vi "Actor Core.vi"(8 "error in":errorcluster, 11 "ListboxBusMonitorPanel in":refnum<class "ListboxBusMonitorPanel.lvclass">) -> (0 "error out":errorcluster, 3 "Actor out":refnum<class "Actor.lvclass">)   [LabVIEW 2020, in "MVA Framework.lvlib" / "ListboxBusMonitor.lvlib" / "ListboxBusMonitorPanel.lvclass"]
doc: "(<B>Filename</B>: Actor Framework.lvlib:Actor.lvclass:Actor Core.vi)\n\nReceives messages to the actor, reacts to them, and initiates any error handling that may shut the actor down.\n\nDescendant classes may override this VI to append parallel tasks for the actor to complete while it handles messages. Overrides use the Call Parent Method node."
uses:
  ListboxBusMonitorPanel.lvclass
  <vilib>/ActorFramework/Actor/Actor.lvclass
  ListboxBusMonitorPanel.lvclass/ListboxBusMonitorPanel.ctl
  modules/listbox-extensions/Source/ListboxExtensions.lvlib
panel:
  in  "Multicolumn Listbox":i32(listbox)
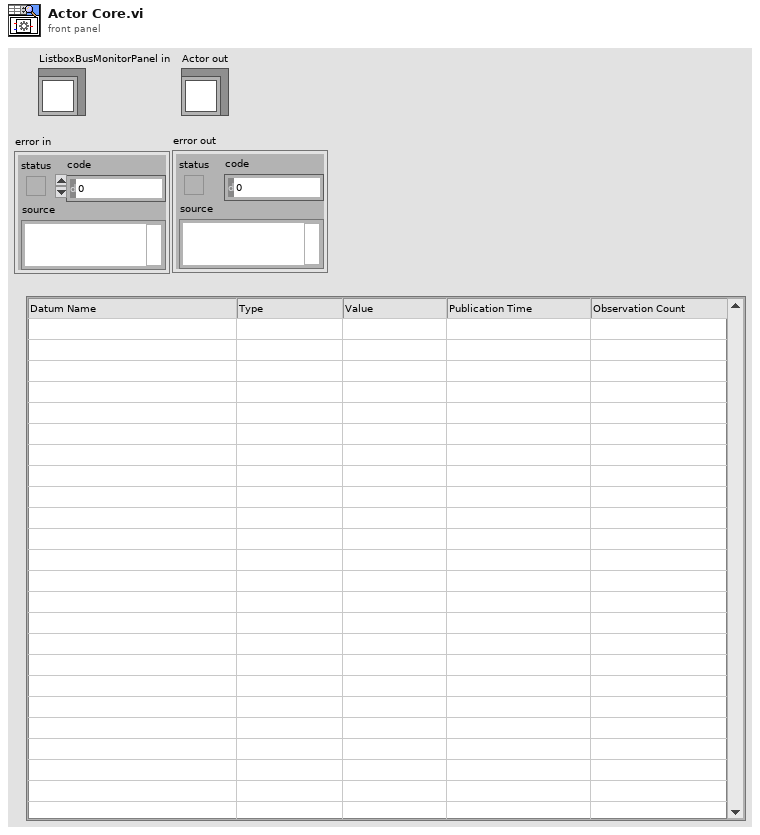
[diagram p1: front panel]
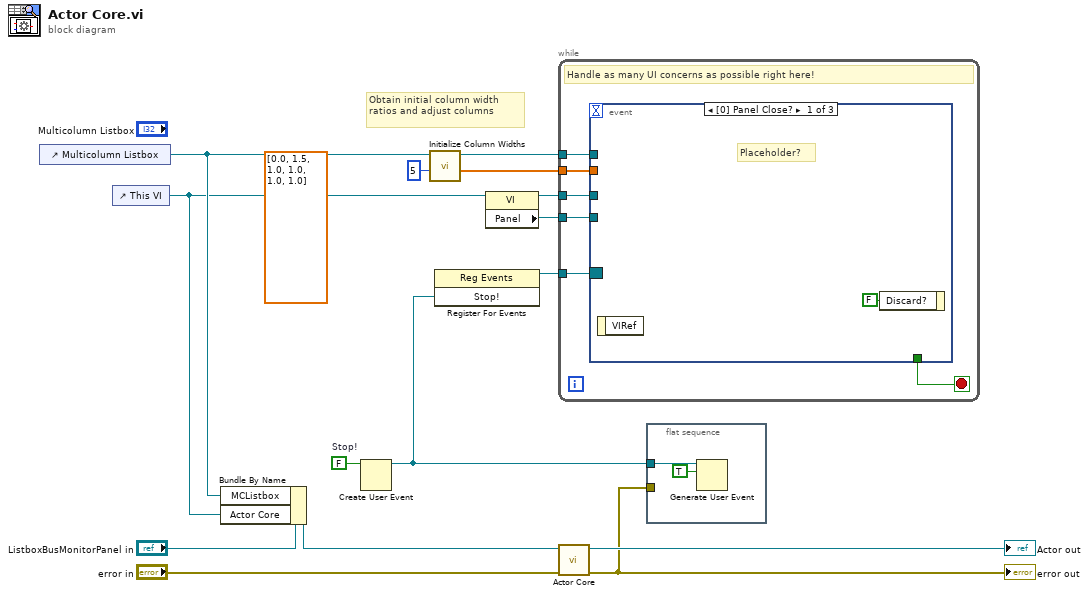
[diagram p0: block diagram]
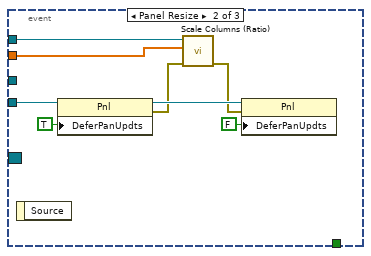
[diagram p2: hidden frame]
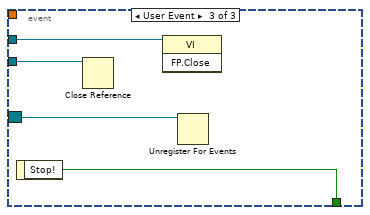
[diagram p3: hidden frame]
diagram:
  (unwired) dbl[] [0.0, 1.5, 1.0, 1.0, 1.0, 1.0] ("Column Widths (Ratio)")
  w10 = FALSE  # Stop!
  # "Obtain initial column width\nratios and adjust columns"
  n1 = control-ref of="Multicolumn Listbox"() -> (w7:refnum<vi>)
  n2 = control-ref of="This VI"() -> (w1:refnum<vi>)
  n3 = Bundle By Name(cluster="ListboxBusMonitorPanel in", "MCListbox"=w7, "Actor Core"=w1) -> (w12:refnum<class "ListboxBusMonitorPanel.lvclass">)
  n4 = Create User Event(user event datatype=w10) -> (user event=w9:refnum<user-event>)  [unwired: 1 in, 1 out]
  n5 = call "Initialize Column Widths.vi"("Number of Columns"=5 ("Number of Columns (including header)"), "MCListbox Reference"=w7) -> ("Column Widths (Ratio)"=w2:dbl[], "MCListbox Reference Out"=w6:refnum<vi>)  [unwired: 8 in]
  n6 = register-events(w9) -> (reference out=w11:refnum<event-registration>)  [unwired: 2 in, 1 out]
  n7 = property class="VI"(reference=w1) -> (reference out=w4:refnum<vi>, "Panel"=w3:refnum<vi>)  [unwired: 1 in, 1 out]
  n8 = while {
    tunnel: w11 -> [w21]
    tunnel: w6 -> [w19]
    tunnel: w2 -> [w18]
    tunnel: w4 -> [w17]
    tunnel: w3 -> [w16]
    stop <- w20 stop-if-true
    # "Handle as many UI concerns as possible right here!"
    n9 = event shown="[0] Panel Close?" {
      selector: w21 -> [_ _ w33]
      dyn-events: _ -> [_ _ _]
      timeout: _ -> [_ _ _]
      tunnel: [_ _ w34] -> w20
      tunnel: w19 -> [_ w29 _]
      tunnel: w18 -> [_ w28 _]
      tunnel: w17 -> [_ _ w32]
      tunnel: w16 -> [_ w27 w31]
      event Panel Close? {
        # "Placeholder?"
        n10 = event-data() -> ()  [unwired: 1 in, 1 out]
        n11 = event-data("Discard?"=FALSE) -> ()  [unwired: 1 in, 1 out]
      }
      event Panel Resize {
        n12 = event-data() -> ()  [unwired: 1 in, 1 out]
        n13 = property class="Pnl"(reference=w27, "DeferPanUpdts"=TRUE ("Defer Panel Updates")) -> (reference out=w30:refnum<vi>, error out=w25:errorcluster)  [unwired: 1 in]
        n14 = call "Scale Columns (Ratio).vi"("error in (no error)"=w25, "Column Widths [unitless ratio]"=w28, "MulticolumnListbox in"=w29) -> ("error out"=w23:errorcluster)  [unwired: 8 in]
        n15 = property class="Pnl"(reference=w30, error in=w23, "DeferPanUpdts"=FALSE ("Defer Panel Updates")) -> ()  [unwired: 2 out]
      }
      event User Event {
        n16 = event-data() -> ("Stop!"=w34:bool)  [unwired: 1 in]
        n17 = Close Reference(reference=w31) -> ()  [unwired: 1 in, 1 out]
        n18 = invoke class="VI" method="FP.Close"(reference=w32) -> ()  [unwired: 2 in, 3 out]
        n19 = Unregister For Events(event registration refnum=w33) -> ()  [unwired: 1 in, 1 out]
      }
    }
  }
  n20 = call-parent "Actor Core.vi"("error in"="error in", "Actor in"=w12) -> ("error out"=w8:errorcluster, "Actor out"=→"Actor out":refnum<class "Actor.lvclass">)  [unwired: 8 in]
  "error out" <- w8
  n21 = flat-sequence {
    tunnel: w9 -> [w36]
    tunnel: w8 -> [_]
    frame #0 {
      n22 = Generate User Event(user event=w36, event data cluster=TRUE ("event data")) -> ()  [unwired: 2 in, 2 out]
    }
  }
